vi "DataTreeCtrl loadData.vi"(8 "error in (no error)":errorcluster, 11 "DataTreeCtrl in":refnum<class "DataTreeCtrl.lvclass">) -> (0 "error out":errorcluster, 2 "signalMultiData":waveform(sgl)[](array[waveform]), 3 "DataTreeCtrl out":refnum<class "DataTreeCtrl.lvclass">)   [LabVIEW 2018, in "DataTreeCtrl.lvclass"]
uses:
  DataTreeCtrl.lvclass
  <vilib>/Utility/miscctls.llb/LVRowAndColumnUnsignedTypeDef.ctl
  DataTreeCtrl.lvclass/DataTreeCtrl.ctl
  ctl/FMstateMachineEnum.ctl
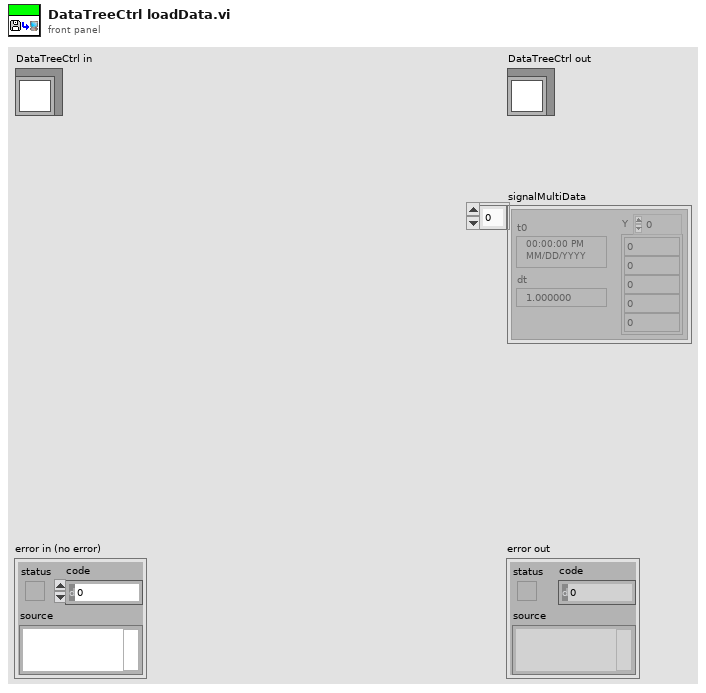
[diagram p1: front panel]
types:
  T1 = typedef "LVRowAndColumnUnsignedTypeDef.ctl" = cluster{"Row":u32, "Column":u32}
  T2 = typedef "FMstateMachineEnum.ctl" = enum16{"none", "init", "openTDMS", "closeTDMS", "getDataList", "getDataInfo", "getTimeStamp", "getCurrPath", "getRemark", "overwriteRemark", "readData", "deleteData", "moveData"}
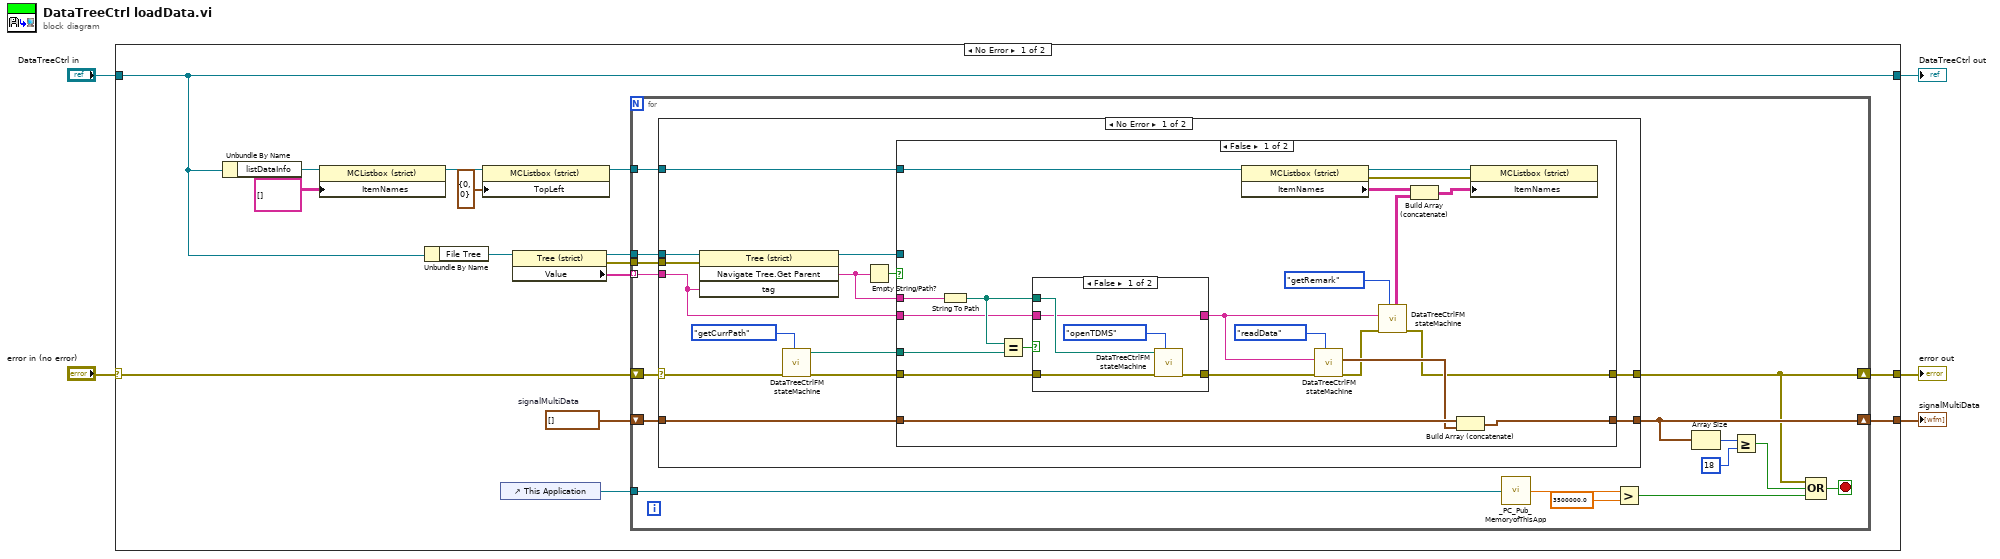
[diagram p0: block diagram]
diagram:
  n1 = case shown="No Error" "error in (no error)" {
    selector: "error in (no error)" -> [w12 w84]
    tunnel: [w16 w84] -> w4
    tunnel: [w11 w83] -> w2
    tunnel: "DataTreeCtrl in" -> [w11 w83]
    tunnel: [w14 _] -> w1
    frame No Error {
      w15 = waveform(sgl)[] []  # signalMultiData
      n2 = Unbundle By Name(w11) -> ("listDataInfo"=w10:refnum<vi>)
      n3 = property class="MCListbox (strict)"(reference=w10, "ItemNames"=string[][] [] ("Item Names")) -> (reference out=w8:refnum<vi>)  [unwired: 1 in, 1 out]
      n4 = Unbundle By Name(w11) -> ("File Tree"=w20:refnum<vi>)
      n5 = property class="MCListbox (strict)"(reference=w8, "TopLeft"=T1 {"Row"=0, "Column"=0} ("Top Left Visible Cell")) -> (reference out=w7:refnum<vi>)  [unwired: 1 in, 1 out]
      n6 = control-ref of="This Application"() -> (w13:refnum<vi>)
      n7 = property class="Tree (strict)"(reference=w20) -> (reference out=w18:refnum<vi>, error out=w17:errorcluster, "Value"=w19:string[])  [unwired: 1 in]
      n8 = for {
        tunnel: w19 -> [w31] mode=indexing
        tunnel: w18 -> [w36]
        tunnel: w17 -> [w35]
        shift-right: [w22] -> w16
        shift-left: w12 -> [w32]
        shift-right: [w29] -> w14
        shift-left: w15 -> [w30]
        tunnel: w13 -> [w25]
        tunnel: w7 -> [w21]
        stop <- w26 stop-if-true
        n9 = case shown="No Error" w32 {
          selector: w32 -> [w41 w82]
          tunnel: w36 -> [w50 _]
          tunnel: w35 -> [w49 _]
          tunnel: w31 -> [w43 _]
          tunnel: [w46 w82] -> w22
          tunnel: w30 -> [w45 w81]
          tunnel: [w44 w81] -> w29
          tunnel: w21 -> [w37 _]
          frame No Error {
            n10 = invoke class="Tree (strict)" method="Navigate Tree.Get Parent"(reference=w50, error in=w49, "tag"=w43) -> (reference out=w38:refnum<vi>, "Navigate Tree:Get Parent"=w47:string)  [unwired: 1 in, 2 out]
            n11 = call "DataTreeCtrlFM stateMachine.vi"("Func"=FMstateMachineEnum."getCurrPath", "error in (no error)"=w41) -> ("error out"=w39:errorcluster, "tdmsFilePath out"=w40:path)  [unwired: 4 in, 4 out]
            n12 = Empty String/Path?(string/path=w47) -> (empty?=w48:bool)
            n13 = case shown="False" w48 {
              tunnel: w47 -> [w71 _]
              tunnel: [w57 w80] -> w46
              tunnel: w39 -> [w68 w80]
              tunnel: w45 -> [w64 w79]
              tunnel: [w62 w79] -> w44
              tunnel: w40 -> [w70 _]
              tunnel: w43 -> [w61 _]
              tunnel: w38 -> [_ _]
              tunnel: w37 -> [w56 _]
              frame False {
                n14 = String To Path(string=w71) -> (path=w65:path)
                n15 = Equal?(x=w65, y=w70) -> (x = y?=w69:bool)
                n16 = case shown="False" w69 {
                  tunnel: w61 -> [w72 w77]
                  tunnel: w68 -> [w74 w78]
                  tunnel: [w73 w78] -> w66
                  tunnel: w65 -> [w75 _]
                  tunnel: [w72 w77] -> w58
                  frame False {
                    n17 = call "DataTreeCtrlFM stateMachine.vi"("Func"=FMstateMachineEnum."openTDMS", "error in (no error)"=w74, "tdmsFilePath in"=w75) -> ("error out"=w73:errorcluster)  [unwired: 3 in, 5 out]
                  }
                  frame True {
                  }
                }
                n18 = property class="MCListbox (strict)"(reference=w56) -> (reference out=w55:refnum<vi>, error out=w54:errorcluster, "ItemNames"=w52:string[][])  [unwired: 1 in]
                n19 = call "DataTreeCtrlFM stateMachine.vi"("Func"=FMstateMachineEnum."readData", "error in (no error)"=w66, "singleDataName"=w58) -> ("error out"=w59:errorcluster, "signalData"=w63:waveform(sgl))  [unwired: 3 in, 4 out]
                n20 = call "DataTreeCtrlFM stateMachine.vi"("Func"=FMstateMachineEnum."getRemark", "error in (no error)"=w59, "singleDataName"=w58) -> ("error out"=w57:errorcluster, "outputArr"=w53:string[][])  [unwired: 3 in, 4 out]
                n21 = Build Array (concatenate)(w52, w53) -> (w51:string[][])
                n22 = Build Array (concatenate)(w64, w63) -> (w62:waveform(sgl)[])
                n23 = property class="MCListbox (strict)"(reference=w55, error in=w54, "ItemNames"=w51) -> ()  [unwired: 2 out]
              }
              frame True {
              }
            }
          }
          frame Error {
          }
        }
        n24 = call "_PC_Pub_MemoryofThisApp.vi"("ThisApp Ref"=w25) -> ("number"=w33:dbl)
        n25 = Greater?(x=w33, y=sgl 3500000.0) -> (0:w27:bool)
        n26 = Array Size(array=w29) -> (size(s)=w24:i32)
        n27 = Greater Or Equal?(x=w24, y=18) -> (x >= y?=w28:bool)
        n28 = Compound Arithmetic op=OR(w22, w28, w27) -> (w26:bool)
      }
    }
    frame Error {
    }
  }
  "error out" <- w4
  "DataTreeCtrl out" <- w2
  "signalMultiData" <- w1
